vi "punto5.vi"() -> ()   [LabVIEW 2021]
uses:
  <vilib>/measure/madcrms.llb/Basic Averaged DC-RMS for 1 Chan.vi
  <vilib>/measure/NI_MAPro.lvlib
panel:
  out "Waveform Graph":dynamicdata(graph)
  out "VPP>3V":bool
  out "Amplitude":dbl
  out "Frequency":dbl
  out "Offset":dbl format="%0.2p"
  out "Acquired signal":dynamicdata(graph)
  out "Generated signal":waveform(dbl)(graph)
  out "Array":dbl[](array[numeric])
  out "Single sample":dynamicdata(graph)
  out "Generator samples chart":dynamicdata(graph)
  in  "stop":bool
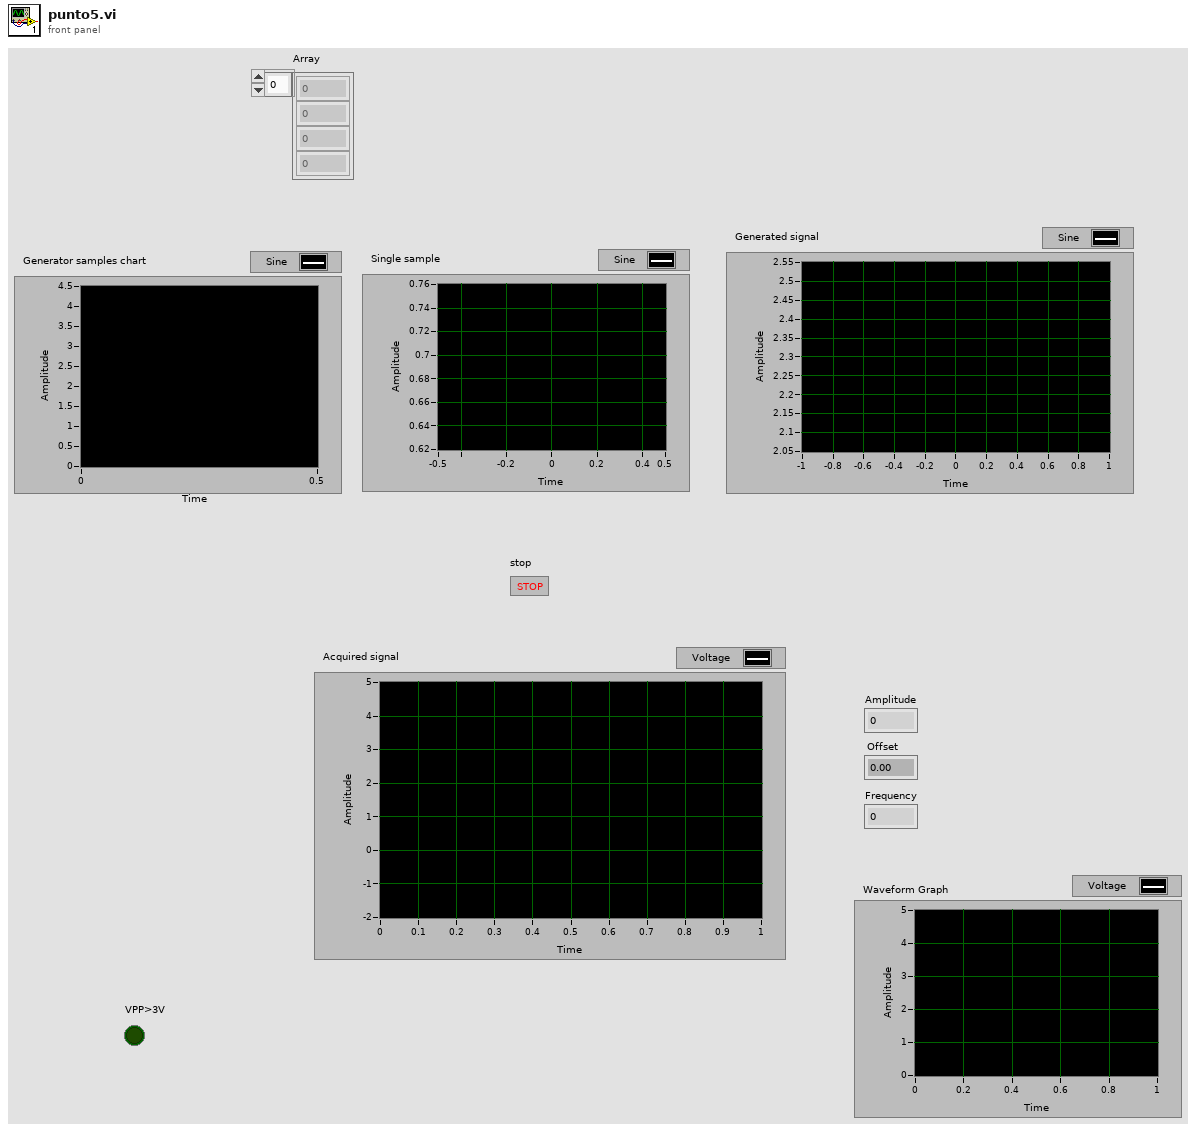
[diagram p1: front panel]
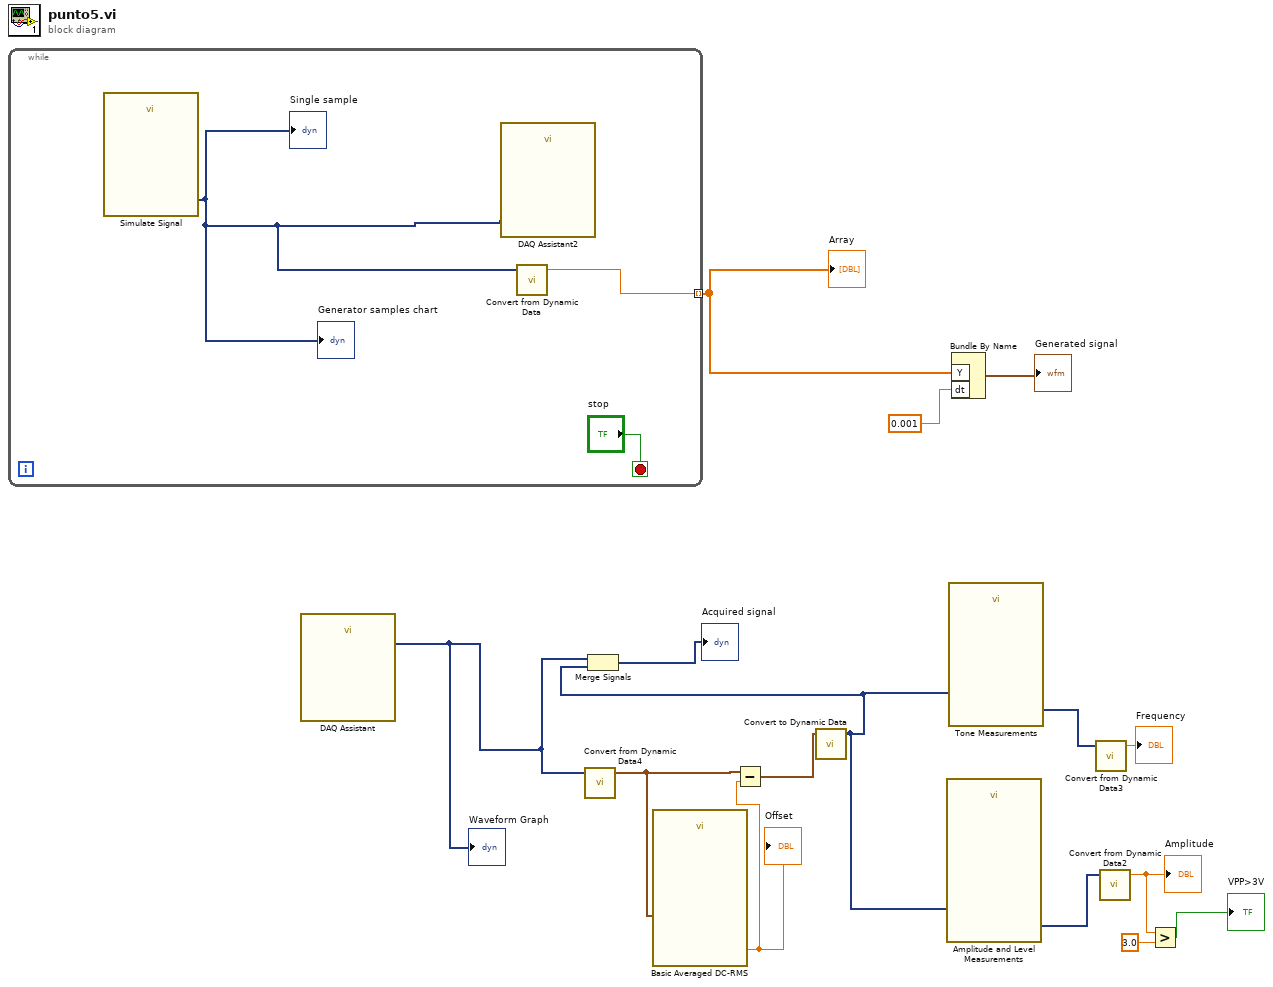
[diagram p0: block diagram]
diagram:
  n1 = while {
    tunnel: [w17] -> w13 mode=indexing
    stop <- "stop" stop-if-true
    n2 = call "Simulate Signal"() -> ("Sine"=w16:dynamicdata)  [unwired: 14 in, 1 out]
    "Generator samples chart" <- w16
    "Single sample" <- w16
    n3 = call "DAQ Assistant2"("data"=w16) -> ()  [unwired: 17 in, 2 out]
    n4 = call "Convert from Dynamic Data"("Dynamic Data Type"=w16) -> ("Scalar"=w17:dbl)  [unwired: 3 in]
  }
  "Array" <- w13
  n5 = call "DAQ Assistant"() -> ("data"=w1:dynamicdata)  [unwired: 17 in, 2 out]
  "Waveform Graph" <- w1
  n6 = call "Convert from Dynamic Data4"("Dynamic Data Type"=w1) -> ("Waveform"=w3:waveform(dbl))  [unwired: 3 in]
  n7 = call-poly <vilib>:"Basic Averaged DC-RMS.vi"("signal in"=w3) -> ("DC value"=w2:dbl)  [unwired: 7 in, 3 out]
  "Offset" <- w2
  n8 = Subtract(x=w3, y=w2) -> (x-y=w11:waveform(dbl))
  n9 = call "Convert to Dynamic Data"("Waveform"=w11) -> ("Dynamic Data Type"=w7:dynamicdata)  [unwired: 3 in]
  n10 = Merge Signals(w1, w7) -> (→"Acquired signal":dynamicdata)
  n11 = call "Amplitude and Level Measurements"("Signals"=w7) -> ("Peak to Peak"=w10:dynamicdata)  [unwired: 13 in, 1 out]
  n12 = call "Tone Measurements"("Signals"=w7) -> ("Frequency"=w9:dynamicdata)  [unwired: 9 in, 1 out]
  n13 = Bundle By Name("Y"=w13, "dt"=0.001) -> (→"Generated signal":waveform(dbl))  [unwired: 1 in]
  n14 = call "Convert from Dynamic Data3"("Dynamic Data Type"=w9) -> ("Scalar"=→"Frequency":dbl)  [unwired: 3 in]
  n15 = call "Convert from Dynamic Data2"("Dynamic Data Type"=w10) -> ("Scalar"=w5:dbl)  [unwired: 3 in]
  "Amplitude" <- w5
  n16 = Greater?(x=w5, y=3.0) -> (0:→"VPP>3V":bool)
